vi "Import Settings.vi"(11 "Settings UI in":refnum<class "Settings UI.lvclass">) -> (3 "Settings UI out":refnum<class "Settings UI.lvclass">)   [LabVIEW 2020, in "Output Sequencer.lvlib" / "Settings UI.lvclass"]
uses:
  Settings UI.lvclass
  Settings UI.lvclass/Settings UI.ctl
  Globals/Dialog Strings.vi
  Output Sequencer/Output Sequencer.lvclass
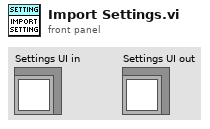
[diagram p1: front panel]
types:
  T1 = typedef "Output Sequencer.lvlib/Settings UI.lvclass/Settings.ctl" = cluster{"Plug-in Version":string, "Step Values":T2[], "Only Execute When Test Running":bool, "Reset Sequence When Test Starts":bool, "Number of Sequence Steps":i32, "Num of Analog Channels":i32, "Num of Digital Channels":i32, "Delay Before Starting Sequence":dbl, "Default Analog Values":dbl[], "Default Digital Values":bool[], "Max Iterations":u32, "Use last value when stopped":bool, "Prioritize exact values":bool, "Enable advanced step timing":bool, "Enable step conditions":bool, "Show confirmation dialogs":bool, "Start condition":string, "Enable re-triggering":bool, "Stop condition":string}
  T2 = typedef "Output Sequencer.lvlib/Settings UI.lvclass/Step Settings.ctl" = cluster{"Description":string, "Precondition":string, "Duration":dbl, "Mode":string, "Delay Between Values":dbl, "Analog Values":string[], "Digital Values":string[], "Postcondition":string, "On True":string, "On False":string}
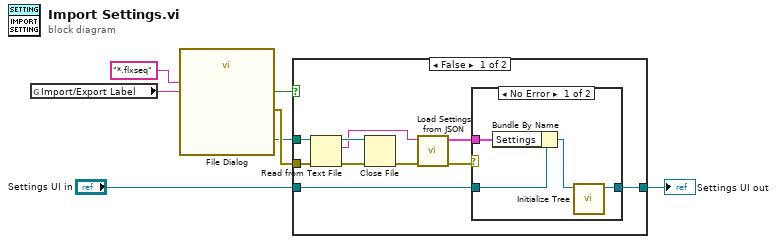
[diagram p0: block diagram]
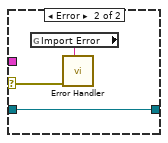
[diagram p2: hidden frame]
diagram:
  n1 = global read "Dialog Strings.vi" "Import/Export Label"() -> (w1:string)
  n2 = call "File Dialog"("pattern (all files)"="*.flxseq", "pattern label"=w1) -> ("selected path"=w2:path, "cancelled"=w3:bool, "error out"=w4:errorcluster)  [unwired: 10 in, 1 out]
  n3 = case shown="False" w3 {
    tunnel: w2 -> [w15 _]
    tunnel: [w11 w25] -> w7
    tunnel: w4 -> [w10 _]
    tunnel: "Settings UI in" -> [w8 w25]
    frame False {
      n4 = Read from Text File(file (use dialog)=w15, error in=w10) -> (refnum out=w17:refnum<file>, text=w13:string, error out=w16:errorcluster)  [unwired: 2 in, 1 out]
      n5 = Close File(refnum=w17, error in=w16) -> (error out=w14:errorcluster)  [unwired: 1 out]
      n6 = call "Load Settings from JSON.vi"("error in (no error)"=w14, "JSON String"=w13) -> ("error out"=w9:errorcluster, "Settings out"=w12:T1)  [unwired: 8 in]
      n7 = case shown="No Error" w9 {
        selector: w9 -> [_ w22]
        tunnel: w12 -> [w20 _]
        tunnel: [w21 w24] -> w11
        tunnel: w8 -> [w19 w24]
        frame No Error {
          n8 = Bundle By Name(cluster=w19, "Settings"=w20) -> (w18:refnum<class "Settings UI.lvclass">)
          n9 = call "Initialize Tree.vi"("UI Data in"=w18) -> ("UI Data out"=w21:refnum<class "Settings UI.lvclass">)  [unwired: 10 in]
        }
        frame Error {
          n10 = global read "Dialog Strings.vi" "Import Error"() -> (w23:string)
          n11 = call "Error Handler.vi"("Dialog Title (\"\")"=w23, "error in (no error)"=w22) -> ()  [unwired: 9 in, 1 out]
        }
      }
    }
    frame True {
    }
  }
  "Settings UI out" <- w7
